vi "HTTP-Check Response Code.vi"(5 "headers":string, 11 "error in":errorcluster, 13 "message":string) -> (15 "error out":errorcluster)   [LabVIEW 2020]
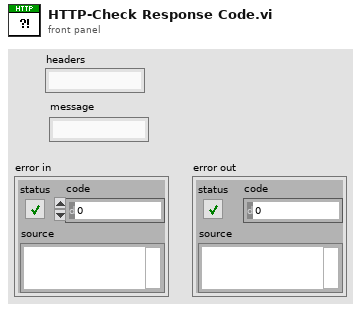
[diagram p1: front panel]
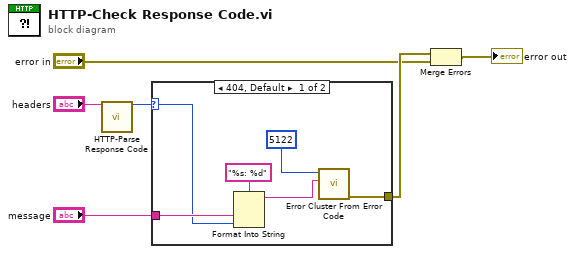
[diagram p0: block diagram]
diagram:
  n1 = call "HTTP-Parse Response Code.vi"("headers"="headers") -> ("code"=w6:i32)  [unwired: 14 in]
  n2 = case shown="404, Default" w6 {
    selector: w6 -> [w10 _]
    tunnel: [w7 _] -> w5
    tunnel: "message" -> [w11 _]
    frame 404, Default {
      n3 = Format Into String(format string="%s: %d", w11, w10) -> (resulting string=w8:string)  [unwired: 2 in, 1 out]
      n4 = call <vilib>:"Error Cluster From Error Code.vi"("error message (\"\")"=w8, "error code (0)"=5122 ("code")) -> ("error out"=w7:errorcluster)  [unwired: 7 in]
    }
    frame 200 {
    }
  }
  n5 = Merge Errors(w5, "error in") -> (→"error out":errorcluster)
